vi "niRFUtil WFM Average (DVR).vi"   [LabVIEW 2015, in "niRFUtil.lvlib"]
doc: "(c) Copyright 2006, National Instruments, Inc. This VI may not be duplicated, sold, or distributed without written consent from National Instruments."
uses:
  niRFUtil.lvlib
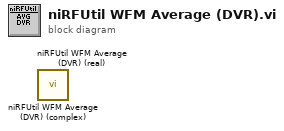
[diagram p0: block diagram]
diagram:
  n1 = call "niRFUtil WFM Average (DVR) (complex).vi"() -> ()  [unwired: 13 in, 3 out]
  n2 = call "niRFUtil WFM Average (DVR) (real).vi"() -> ()  [unwired: 13 in, 3 out]
